vi "To JSON.vi"(7 "Package Folder":path, 8 "error in (no error)":errorcluster, 11 "Package in":refnum<class "Package.lvclass">) -> (0 "error out":errorcluster, 2 "Package JSON":string, 3 "Package out":refnum<class "Package.lvclass">)   [LabVIEW 2020, in "neg-pkg.lvlib" / "Package.lvclass"]
uses:
  Package.lvclass
  Package.lvclass/Package.ctl
  semver/Semver/Semver.lvclass/Semver.ctl
  semver/Semver/Semver.lvclass
  neg_pkgs/negentropicdev/lv-json/JSON/JSON.lvlib
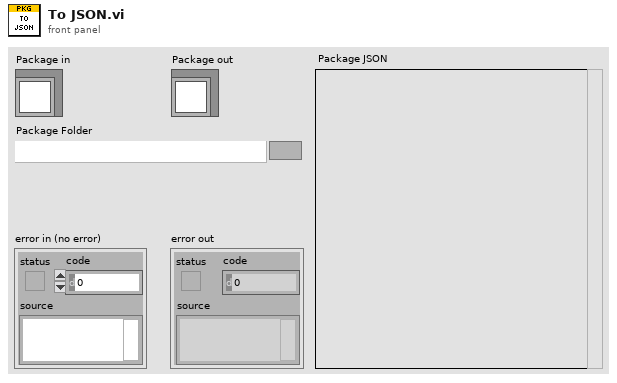
[diagram p1: front panel]
types:
  T1 = typedef "neg-pkg.lvlib/Package.lvclass/Package ID.ctl" = cluster{"Type":T2, "Scope":string, "Name":string, "Resource":string}
  T2 = typedef "neg-pkg.lvlib/Package.lvclass/Package Type.ctl" = enum16{"unspecified", "git"}
  T3 = typedef "neg-pkg.lvlib/Package.lvclass/Dependency.ctl" = cluster{"Package":T1, "Version":string}
  T4 = typedef "neg-pkg.lvlib/Package.lvclass/Build Item.ctl" = cluster{"Project":path, "Target":string, "Build Spec":string}
  T5 = typedef "neg-pkg.lvlib/Package.lvclass/Config Field.ctl" = cluster{"Name":string, "Value":string}
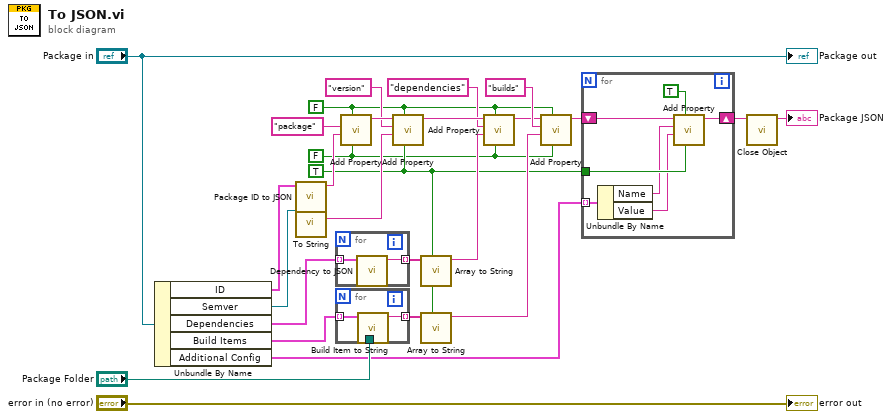
[diagram p0: block diagram]
diagram:
  w1 = FALSE ("String?")
  w8 = FALSE ("Include Empty?")
  w2 = TRUE ("String?")
  n1 = Unbundle By Name("Package in") -> ("ID"=w25:T1, "Semver"=w24:refnum<class "Semver.lvclass">, "Dependencies"=w23:T3[], "Build Items"=w13:T4[], "Additional Config"=w5:T5[])
  n2 = call "Package ID to JSON.vi"("Package"=w25) -> ("Package JSON"=w22:string)  [unwired: 10 in]
  n3 = call "To String.vi"("Semver in"=w24) -> ("Version String"=w19:string)  [unwired: 9 in, 1 out]
  n4 = for {
    tunnel: w23 -> [w29] mode=indexing
    tunnel: [w28] -> w16 mode=indexing
    n5 = call "Dependency to JSON.vi"("Dependency"=w29) -> ("Dependency JSON"=w28:string)  [unwired: 10 in]
  }
  n6 = for {
    tunnel: w13 -> [w32] mode=indexing
    tunnel: "Package Folder" -> [w31]
    tunnel: [w30] -> w11 mode=indexing
    n7 = call "Build Item to String.vi"("Package Folder"=w31, "Build Item"=w32) -> ("String"=w30:string)  [unwired: 9 in]
  }
  n8 = call "Add Property.vi"("String?"=w1, "Include Empty?"=w8, "Value"=w22, "Property Name"="package") -> ("String out"=w20:string)  [unwired: 7 in]
  n9 = call "Add Property.vi"("String?"=w2, "Include Empty?"=w8, "Value"=w19, "Property Name"="version", "String In"=w20) -> ("String out"=w17:string)  [unwired: 6 in]
  n10 = call "Array to String.vi"("Strings? (F)"=w2, "JSON Strings"=w16) -> ("JSON Array String"=w15:string)  [unwired: 9 in]
  n11 = call "Array to String.vi"("Strings? (F)"=w2, "JSON Strings"=w11) -> ("JSON Array String"=w7:string)  [unwired: 9 in]
  n12 = call "Add Property.vi"("String?"=w1, "Include Empty?"=w8, "Value"=w15, "Property Name"="dependencies", "String In"=w17) -> ("String out"=w9:string)  [unwired: 6 in]
  n13 = call "Add Property.vi"("String?"=w1, "Include Empty?"=w8, "Value"=w7, "Property Name"="builds", "String In"=w9) -> ("String out"=w6:string)  [unwired: 6 in]
  n14 = for {
    shift-right: [w33] -> w4
    shift-left: w6 -> [w39]
    tunnel: w2 -> [w37]
    tunnel: w5 -> [w36] mode=indexing
    n15 = Unbundle By Name(w36) -> ("Name"=w35:string, "Value"=w34:string)
    n16 = call "Add Property.vi"("String?"=w37, "Include Empty?"=TRUE, "Value"=w34, "Property Name"=w35, "String In"=w39) -> ("String out"=w33:string)  [unwired: 6 in]
  }
  n17 = call "Close Object.vi"("String In"=w4) -> ("String out"=→"Package JSON":string)  [unwired: 10 in]
  "error out" <- "error in (no error)"
  "Package out" <- "Package in"
